vi "TimerStop.vi"(8 "error in":errorcluster, 10 "millisecond timer start":u32) -> (0 "error out":errorcluster, 2 "millisecond timer difference":u32)   [LabVIEW 2015]
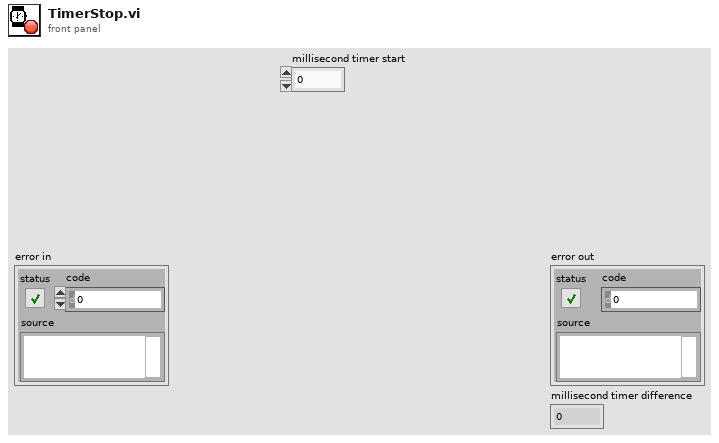
[diagram p1: front panel]
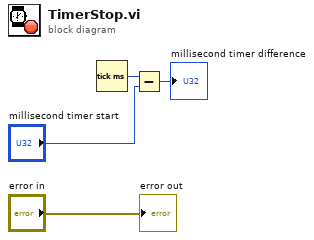
[diagram p0: block diagram]
diagram:
  n1 = Tick Count (ms)() -> (millisecond timer value=w3:u32)
  n2 = Subtract(x=w3, y="millisecond timer start") -> (x-y=→"millisecond timer difference":u32)
  "error out" <- "error in"
